vi "Filter Class Tree_Remove Empty Parent Items.vi"(11 "Array":T1[](array[typedef])) -> (3 "Array":T1[](array[typedef]))   [LabVIEW 2023]
doc: "If parent items is empty after filter actions., remove item."
uses:
  class/Class Item Cluster.ctl
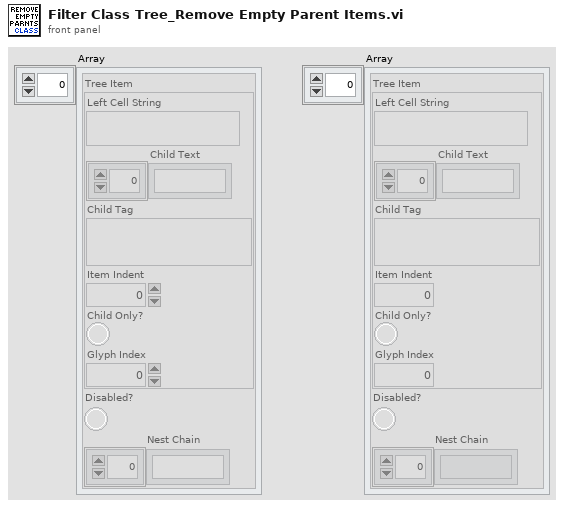
[diagram p1: front panel]
types:
  T1 = typedef "Class Item Cluster.ctl" = cluster{"Tree Item":cluster{"Left Cell String":string, "Child Text":string[], "Child Tag":string, "Item Indent":i32, "Child Only?":bool, "Glyph Index":i32}, "Disabled?":bool, "Nest Chain":string[]}
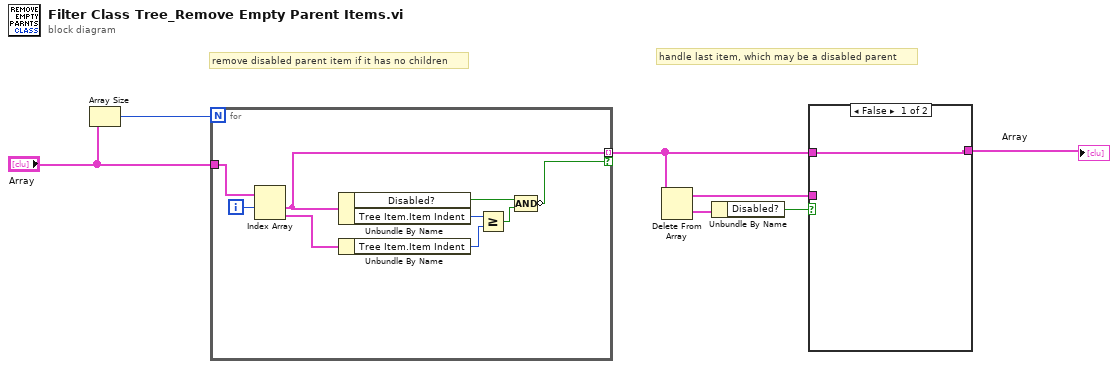
[diagram p0: block diagram]
diagram:
  # "handle last item, which may be a disabled parent"
  # "remove disabled parent item if it has no children"
  n1 = Array Size(array="Array") -> (size(s)=w1:i32)
  n2 = for {
    N: w1 -> [_]
    tunnel: "Array" -> [w8]
    tunnel: [w9] -> w2 mode=indexing if=w10
    i -> [w16]
    n3 = Index Array(array=w8, index #1=w16) -> (element #1=w9:T1, element #2=w15:T1)  [unwired: 1 in]
    n4 = Unbundle By Name(w9) -> ("Disabled?"=w12:bool, "Tree Item.Item Indent"=w14:i32)
    n5 = Unbundle By Name(w15) -> ("Tree Item.Item Indent"=w13:i32)
    n6 = Greater Or Equal?(x=w14, y=w13) -> (x >= y?=w11:bool)
    n7 = Compound Arithmetic op=AND(w12, w11) -> (invert w10:bool)
  }
  n8 = Delete From Array(array=w2) -> (deleted portion=w6:T1, array with subset deleted=w3:T1[])  [unwired: 2 in]
  n9 = Unbundle By Name(w6) -> ("Disabled?"=w5:bool)
  n10 = case shown="False" w5 {
    tunnel: [w17 w18] -> w4
    tunnel: w3 -> [_ w18]
    tunnel: w2 -> [w17 _]
    frame False {
    }
    frame True {
    }
  }
  "Array" <- w4
